vi "nRF24 communication.vi"(8 "error in (no error)":errorcluster) -> (0 "error out":errorcluster)   [LabVIEW 2016]
uses:
  Typedef/Remote Control Cluster.ctl
  Typedef/INS Data.ctl
  Shared resoruces/ODrive State and Info.vi
  Shared resoruces/Navigation Variables.vi
  Shared resoruces/Shared resources RT.lvlib
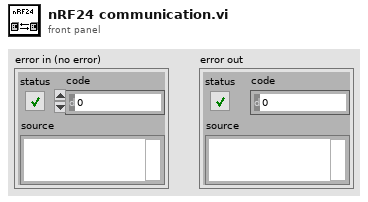
[diagram p1: front panel]
types:
  T1 = typedef "Semaphore RefNum" = refnum<k1>
  T2 = typedef "INS Data.ctl" = cluster{"Yaw":sgl, "Pitch":sgl, "Roll":sgl, "Lat":dbl, "Long":dbl, "Alt":dbl, "North":dbl, "East":dbl, "Down":dbl, "PosU":dbl, "VelU":dbl}
  T3 = typedef "Remote Control Cluster.ctl" = cluster{"Pot1":u16, "Pot2":u16, "Pot3":u16, "Pot4":u16, "Switch1":cluster{"L":bool, "H":bool}, "Switch2":cluster{"L":bool, "H":bool}, "Switch3":cluster{"L":bool, "H":bool}}
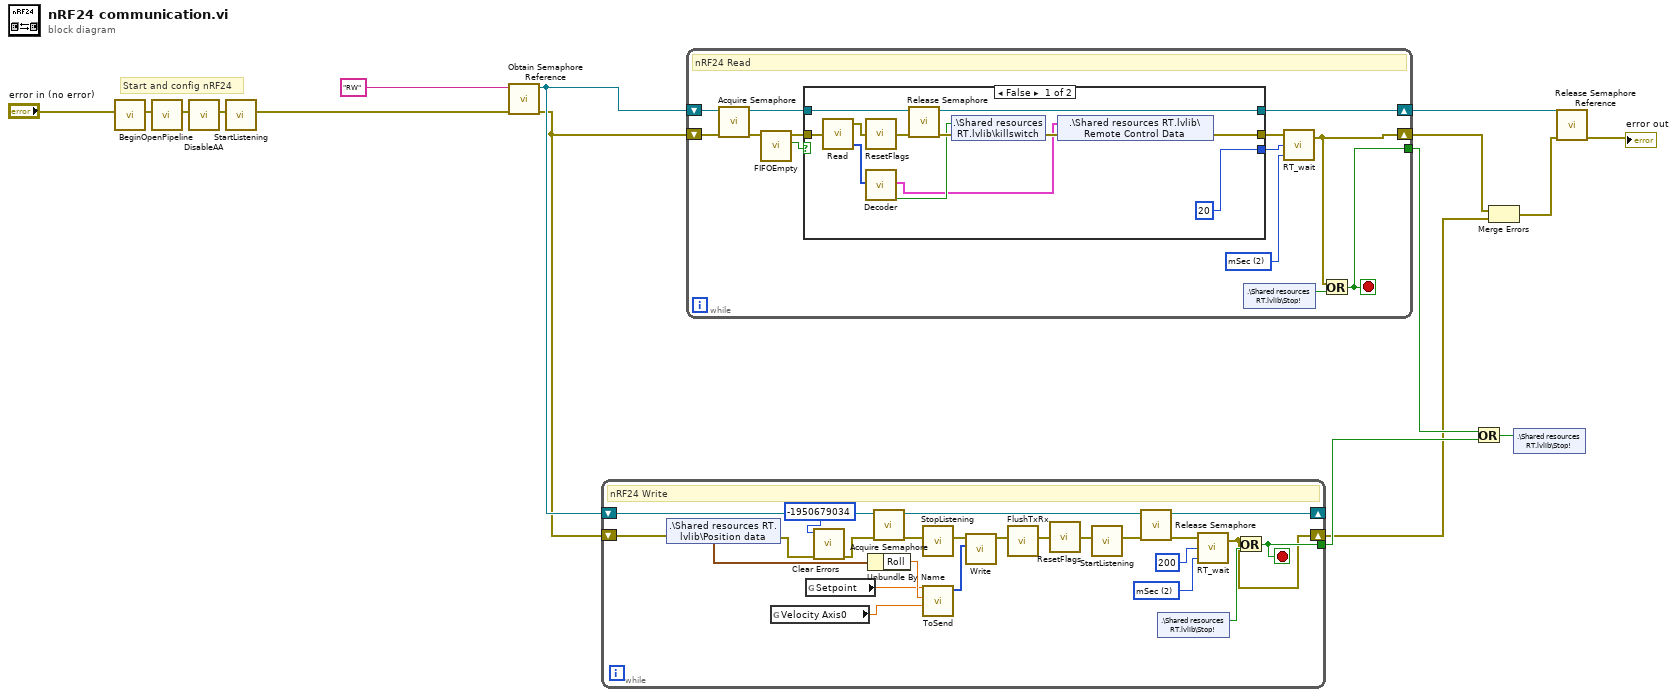
[diagram p0: block diagram]
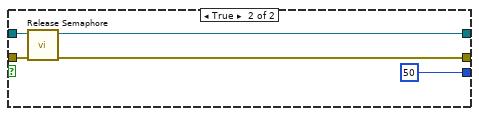
[diagram p2: hidden frame]
diagram:
  # "Start and config nRF24"
  n1 = call "Begin.vi"("error in (no error)"="error in (no error)") -> ("error out"=w2:errorcluster)  [unwired: 10 in]
  n2 = call "OpenPipeline.vi"("error in (no error)"=w2) -> ("error out"=w3:errorcluster)  [unwired: 10 in]
  n3 = call "DisableAA.vi"("error in (no error)"=w3) -> ("error out"=w4:errorcluster)  [unwired: 10 in]
  n4 = call "StartListening.vi"("error in (no error)"=w4) -> ("error out"=w5:errorcluster)  [unwired: 10 in]
  n5 = call <vilib>:"Obtain Semaphore Reference.vi"("error in (no error)"=w5, "name (unnamed)"="RW") -> ("error out"=w7:errorcluster, "semaphore"=w8:T1)  [unwired: 3 in, 1 out]
  n6 = while {
    shift-right: [w34] -> _
    shift-left: w8 -> [w40]
    shift-right: [w17] -> w10
    shift-left: w7 -> [w23]
    tunnel: [w25] -> w14
    stop <- w25 stop-if-true
    w31 = u16 2 items=["Ticks", "uSec", "mSec"] ("Counter Units")
    # "nRF24 Write"
    n7 = shared-variable ".\\Shared resources RT.lvlib\\Position data"(error in=w23) -> (w24:T2, error out=w22:errorcluster)
    n8 = global read "ODrive State and Info.vi" "Velocity Axis0"() -> (w18:dbl)
    n9 = global read "Navigation Variables.vi" "Setpoint"() -> (w19:dbl)
    n10 = call <vilib>:"Clear Errors.vi"("error in (no error)"=w22, "specific error code to clear (0: all)"=-1950679034) -> ("error out"=w21:errorcluster)  [unwired: 4 in, 1 out]
    n11 = Unbundle By Name(w24) -> ("Roll"=w30:sgl)
    n12 = call <vilib>:"Acquire Semaphore.vi"("error in (no error)"=w21, "semaphore"=w40) -> ("error out"=w39:errorcluster, "semaphore out"=w35:T1)  [unwired: 3 in, 1 out]
    n13 = call "StopListening.vi"("error in (no error)"=w39) -> ("error out"=w29:errorcluster)  [unwired: 10 in]
    n14 = call "ToSend.vi"("velocity"=w18, "leanAngel"=w30, "setpoint"=w19) -> ("data2nRF24"=w27:u8[])  [unwired: 8 in]
    n15 = call "Write.vi"("Input"=w27, "error in (no error)"=w29) -> ("error out"=w28:errorcluster)  [unwired: 8 in, 1 out]
    n16 = call "FlushTxRx.vi"("error in (no error)"=w28) -> ("error out"=w38:errorcluster)  [unwired: 10 in]
    n17 = call "ResetFlags.vi"("error in (no error)"=w38) -> ("error out"=w37:errorcluster)
    n18 = call "StartListening.vi"("error in (no error)"=w37) -> ("error out"=w36:errorcluster)  [unwired: 10 in]
    n19 = call <vilib>:"Release Semaphore.vi"("error in (no error)"=w36, "semaphore"=w35) -> ("error out"=w33:errorcluster, "semaphore out"=w34:T1)  [unwired: 4 in]
    n20 = shared-variable ".\\Shared resources RT.lvlib\\Stop!"() -> (w26:bool)  [unwired: 1 in, 1 out]
    n21 = call "RT_wait.vi"("Counter Units"=w31, "Count(mSec)"=u32 200 ("Count(uSec)"), "error in (no error)"=w33) -> ("error out"=w17:errorcluster)  [unwired: 1 in, 1 out]
    n22 = Or(x=w17, y=w26) -> (x .or. y?=w25:bool)
  }
  n23 = while {
    shift-right: [w48] -> w9
    shift-left: w8 -> [w53]
    shift-right: [w42] -> w11
    shift-left: w7 -> [w52]
    tunnel: [w41] -> w15
    stop <- w41 stop-if-true
    w45 = u16 2 items=["Ticks", "uSec", "mSec"] ("Counter Units")
    # "nRF24 Read"
    n24 = call <vilib>:"Acquire Semaphore.vi"("error in (no error)"=w52, "semaphore"=w53) -> ("error out"=w51:errorcluster, "semaphore out"=w49:T1)  [unwired: 3 in, 1 out]
    n25 = call "FIFOEmpty.vi"("error in (no error)"=w51) -> ("RX_EMPTY"=w47:bool, "error out"=w50:errorcluster)  [unwired: 9 in]
    n26 = case shown="False" w47 {
      tunnel: w50 -> [w65 w70]
      tunnel: w49 -> [w62 w69]
      tunnel: [w54 w67] -> w46
      tunnel: [w61 w68] -> w48
      tunnel: [u32 20 ("Count(uSec)") u32 50 ("Count(uSec)")] -> w44
      frame False {
        n27 = call "Read.vi"("error in (no error)"=w65) -> ("error out"=w64:errorcluster, "Data frame"=w60:u16[])  [unwired: 1 out]
        n28 = call "ResetFlags.vi"("error in (no error)"=w64) -> ("error out"=w63:errorcluster)
        n29 = call "Decoder.vi"("Data frame"=w60) -> ("output cluster"=w55:T3, "Kill Switch"=w57:bool)  [unwired: 17 in]
        n30 = call <vilib>:"Release Semaphore.vi"("error in (no error)"=w63, "semaphore"=w62) -> ("error out"=w58:errorcluster, "semaphore out"=w61:T1)  [unwired: 4 in]
        n31 = shared-variable ".\\Shared resources RT.lvlib\\killswitch"(w57, error in=w58) -> (error out=w56:errorcluster)
        n32 = shared-variable ".\\Shared resources RT.lvlib\\Remote Control Data"(w55, error in=w56) -> (error out=w54:errorcluster)
      }
      frame True {
        n33 = call <vilib>:"Release Semaphore.vi"("error in (no error)"=w70, "semaphore"=w69) -> ("error out"=w67:errorcluster, "semaphore out"=w68:T1)  [unwired: 4 in]
      }
    }
    n34 = shared-variable ".\\Shared resources RT.lvlib\\Stop!"() -> (w43:bool)  [unwired: 1 in, 1 out]
    n35 = call "RT_wait.vi"("Counter Units"=w45, "Count(mSec)"=w44, "error in (no error)"=w46) -> ("error out"=w42:errorcluster)  [unwired: 1 in, 1 out]
    n36 = Or(x=w42, y=w43) -> (x .or. y?=w41:bool)
  }
  n37 = Or(x=w15, y=w14) -> (x .or. y?=w13:bool)
  n38 = Merge Errors(w11, w10) -> (w12:errorcluster)
  n39 = shared-variable ".\\Shared resources RT.lvlib\\Stop!"(w13) -> ()  [unwired: 1 in, 1 out]
  n40 = call <vilib>:"Release Semaphore Reference.vi"("error in (no error)"=w12, "semaphore"=w9) -> ("error out"=→"error out":errorcluster)  [unwired: 8 in, 1 out]
